vi "Exemple_Kernel_App_RBFSampler.vi"() -> ()   [LabVIEW 2020]
uses:
  Objet/6 - Datasets Transformation/6.7 - Kernel Approximation/RBFSampler/RBFSampler.lvclass
panel:
  in  "y":string[][](array[string])
  out "error out":errorcluster caption="sortie d'erreur"
  out "Data":T1
  in  "RBFSampler":T2={"gamma"=1.0, "n_components"=100, "random_state"=-1} {"random_state" min=-1}
  in  "error in":errorcluster caption="entrée d'erreur"
  in  "X":string[][](array[string])=[["0", "0"], ["1", "1"], ["1", "0"], ["0", "1"]]
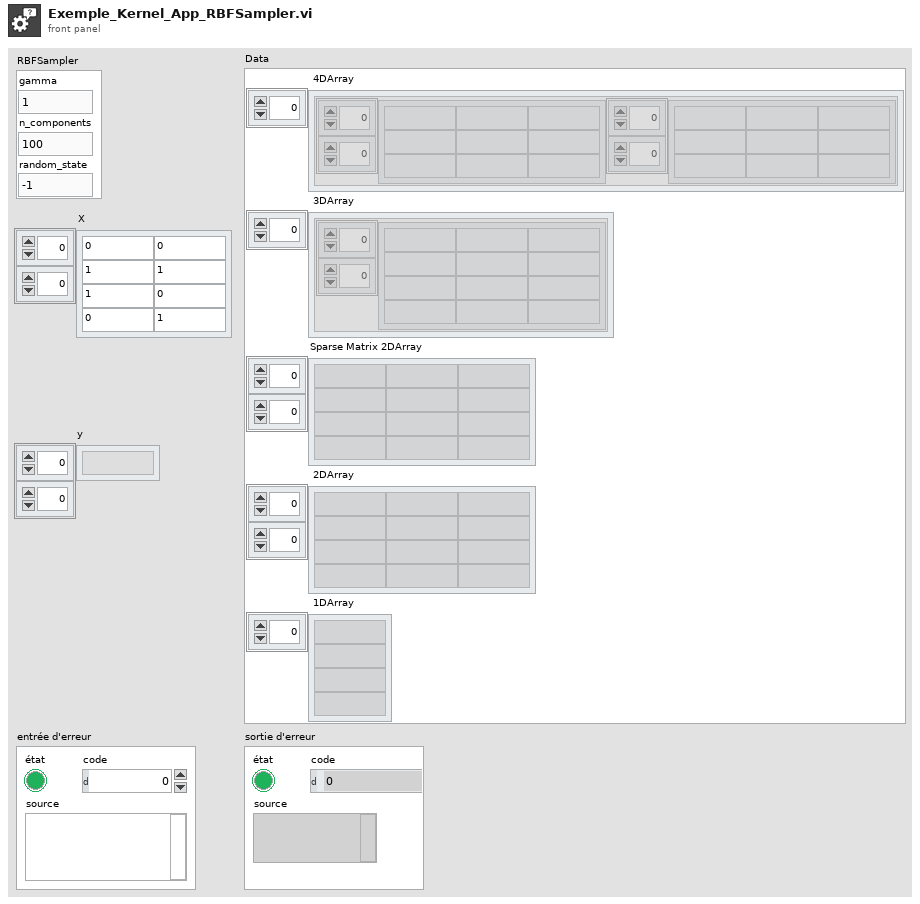
[diagram p1: front panel]
types:
  T1 = cluster{" 4DArray":cluster{"1":string[][], "2":string[][]}[], " 3DArray":cluster{"Tableau":string[][]}[], "Sparse Matrix 2DArray":string[][], " 2DArray":string[][], " 1DArray":string[]}
  T2 = cluster{"gamma":dbl, "n_components":i32, "random_state":i32}
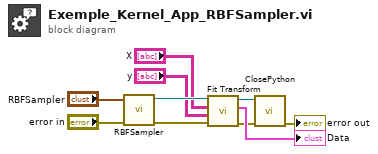
[diagram p0: block diagram]
diagram:
  n1 = call "RBFSampler.vi"("error in"="error in", "RBFSampler"="RBFSampler") -> ("error out"=w7:errorcluster, "RBFSampler.lvclass"=w6:refnum<class "RBFSampler.lvclass">)  [unwired: 8 in]
  n2 = call-dynamic "Fit Transform.vi"("error in (no error)"=w7, "y"="y", "X"="X", "RBFSampler.lvclass"=w6) -> ("error out"=w1:errorcluster, "Data"=→"Data":T1, "RBFSampler.lvclass"=w3:refnum<class "RBFSampler.lvclass">)  [unwired: 5 in]
  n3 = call-dynamic "ClosePython.vi"("error in (no error)"=w1, "Scikit-learn en entrée"=w3) -> ("error out"=→"error out":errorcluster)  [unwired: 8 in, 1 out]
